vi "ESP Set and Get (SubVI).vi"(0 "ESP Config":T1={"COM Port Input"="COM8", "Manual Command"={"Device Type"="", "Instance"="", "Command"="", "Sub-Command"="", "Parameters (Seperate by :)"=""}, "Device Type"="e", "Instance"="a", "Use Manual Command"=TRUE, "Timeout [msec]"=1000, "Read/Write Wait [msec]"=25}, 5 "SET Table Ref":refnum<vi>, 7 "SET-GET Commands Ref":refnum<vi>) -> (4 "ESP Output":T2={"Write Command"="ea:DU:1", "Read String"="\u0006\u0001ea:00.000:00.000:00.036:00.004:AEA8\u0004", "Read Bytes"=12, "Bytes at Port"=12, "Response"="ea:00.000:00.000:00.036:00.004:AEA8", "ACK"=TRUE, "EOT"=TRUE, "NAK"=FALSE, "Parameters"=["00.000", "00.000", "00.036", "00.004"]}, 15 "ESP Error":errorcluster={"status"=FALSE, "code"=1073676294, "source"="VISA Read in ESP-D Read-Write (SubVI).vi->IO Board Evaluate.vi"})   [LabVIEW 2011]
panel:
  out "Error Output":errorcluster
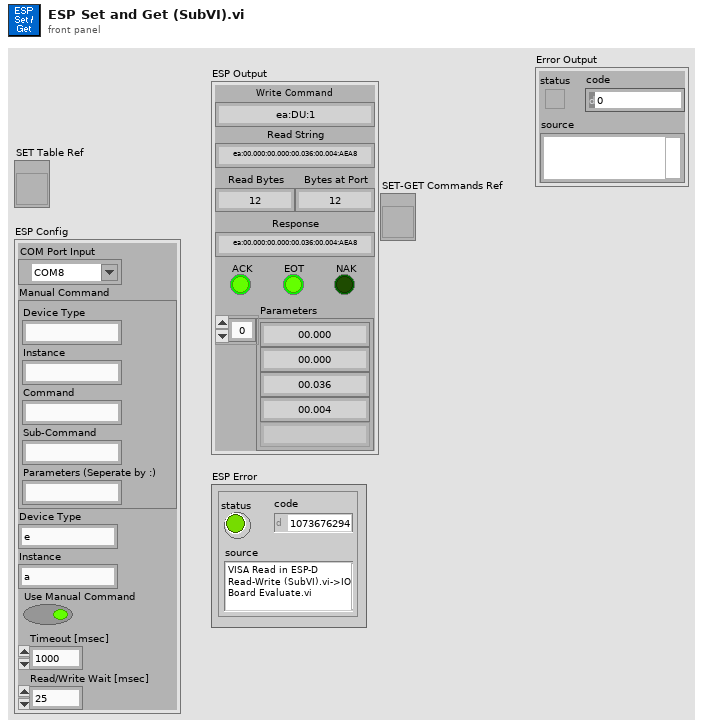
[diagram p1: front panel]
types:
  T1 = cluster{"COM Port Input":refnum<visa-resource-name>, "Manual Command":cluster{"Device Type":string, "Instance":string, "Command":string, "Sub-Command":string, "Parameters (Seperate by :)":string}, "Device Type":string, "Instance":string, "Use Manual Command":bool, "Timeout [msec]":u32, "Read/Write Wait [msec]":u32}
  T2 = cluster{"Write Command":string, "Read String":string, "Read Bytes":u32, "Bytes at Port":u32, "Response":string, "ACK":bool, "EOT":bool, "NAK":bool, "Parameters":string[]}
  T3 = cluster{"Device Type":string, "Instance":string, "Command":string, "Sub-Command":string, "Parameters (Seperate by :)":string}
  T4 = cluster{"CMD_Desc":string, "Param_Names":string[], "Param_Values":string[], "GET":bool, "SET":bool}
  T5 = cluster{"CMD_Desc":string, "Param_Names":string[], "Param_Values":string[], "SET":bool, "GET":bool}[]
  T6 = cluster{"CMD_Desc":string, "Param_Names":string[], "Param_Values":string[], "SET":bool, "GET":bool}
  T7 = cluster{"CMD_Desc":string, "Param_Names":string[], "Param_Values":string[], "GET":bool, "SET":bool}[]
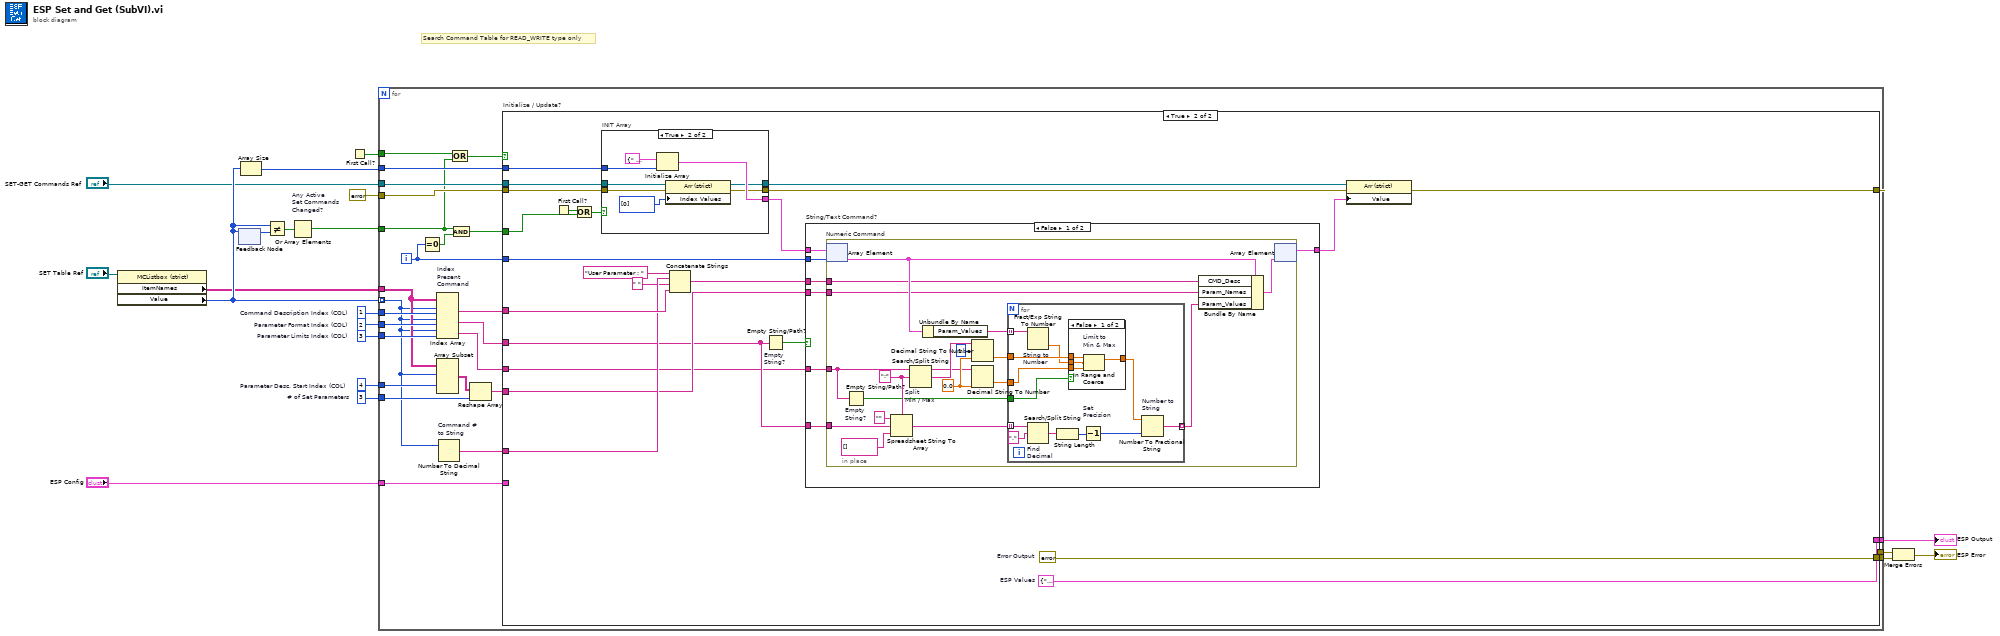
[diagram p0: block diagram]
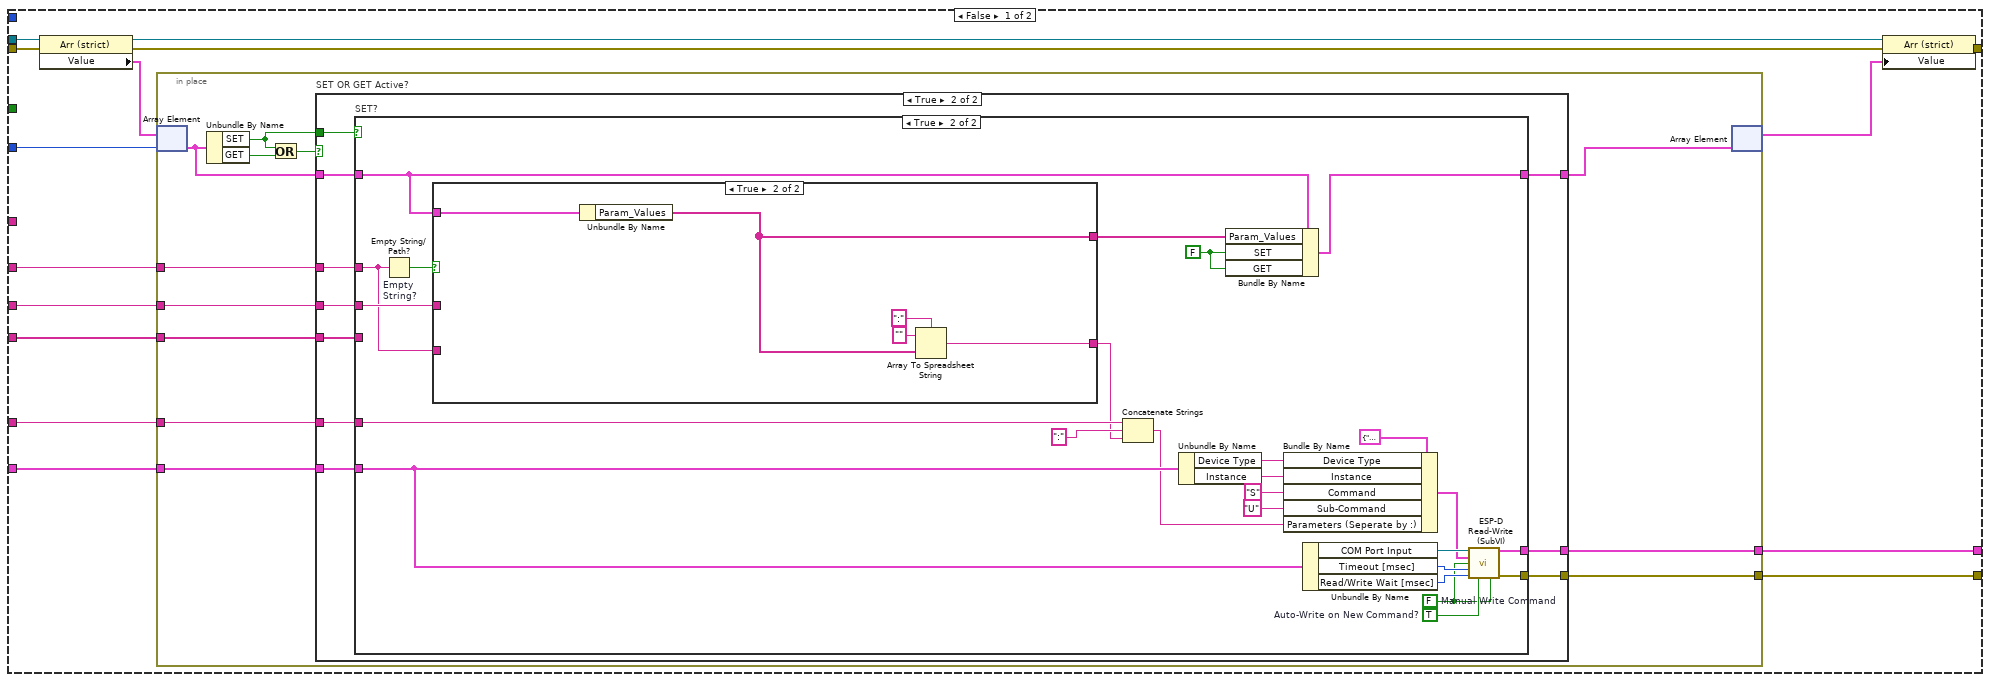
[diagram p2: hidden frame]
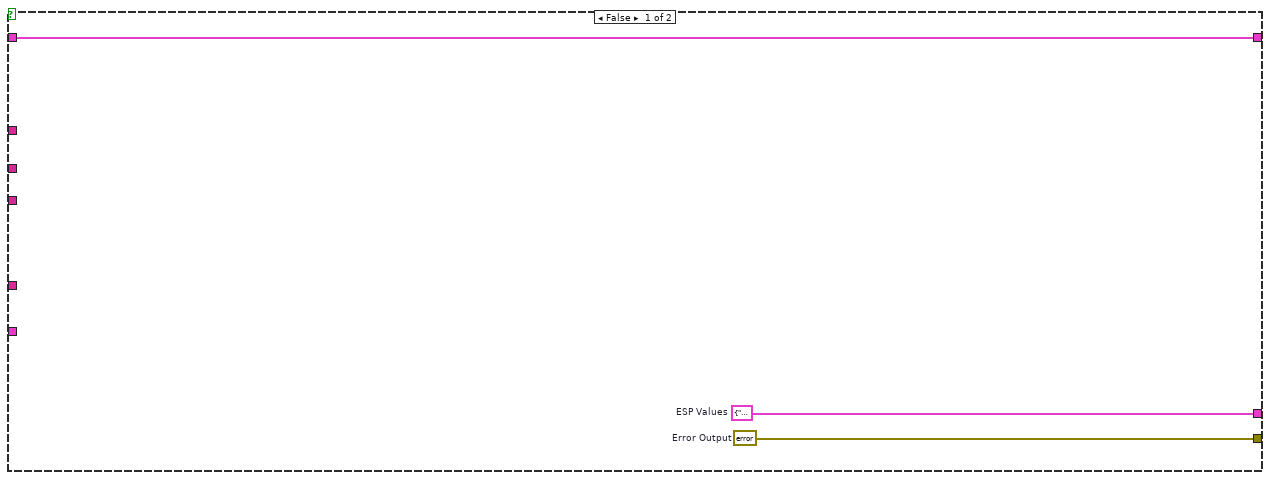
[diagram p3: hidden frame]
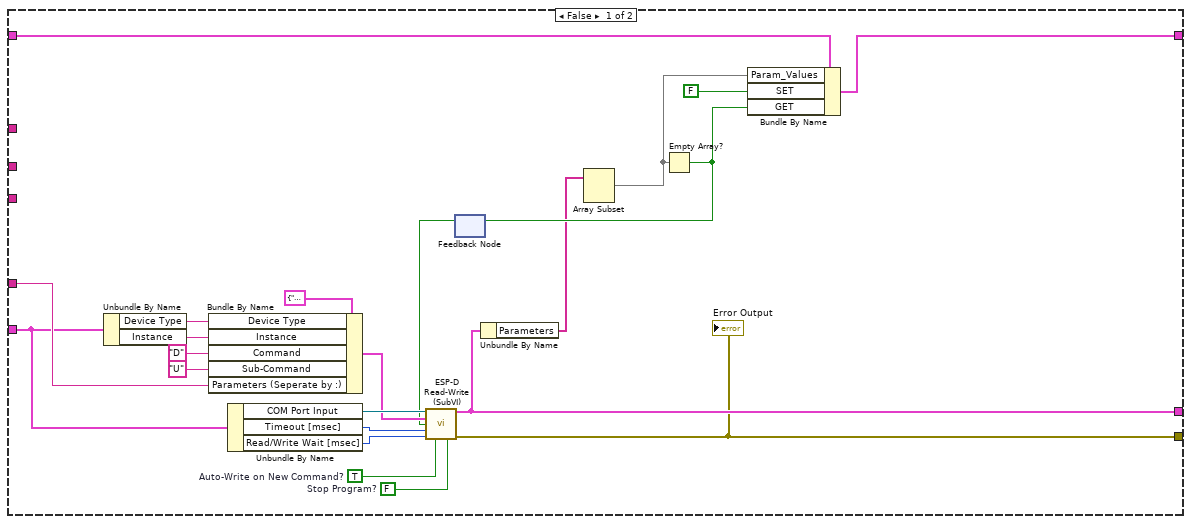
[diagram p4: hidden frame]
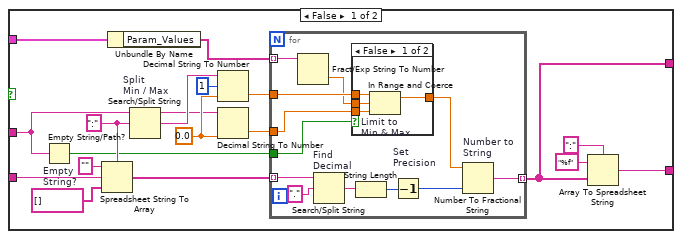
[diagram p5: hidden frame]
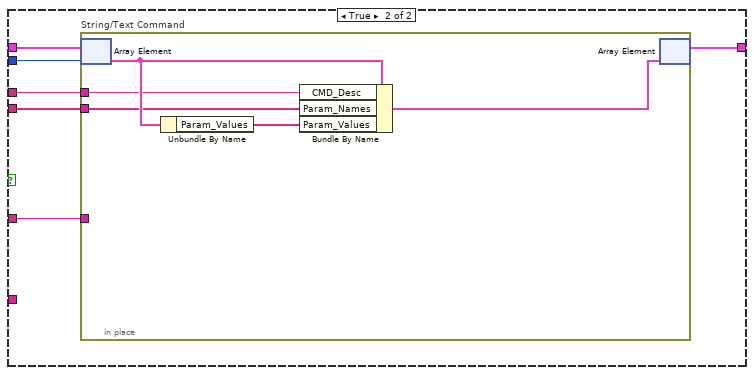
[diagram p8: hidden frame]
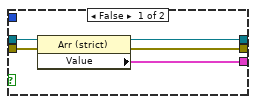
[diagram p9: hidden frame]
diagram:
  w8 = 1  # Command Description Index (COL)
  w5 = 3  # # of Set Parameters
  w6 = 4  # Parameter Desc. Start Index (COL)
  w4 = 3  # Parameter Limits Index (COL)
  w3 = 2  # Parameter Format Index (COL)
  # "Search Command Table for READ_WRITE type only"
  n1 = property class="MCListbox (strict)"(reference="SET Table Ref") -> ("ItemNames"=w9:string[][], "Value"=w14:i32[])  [unwired: 1 in, 2 out]
  n2 = feedback #1() -> (w13:i32[])  [unwired: 1 in]
  n3 = feedback-in #1(w14) -> ()
  n4 = Array Size(array=w14) -> (size(s)=w10:i32)
  n5 = Not Equal?(x=w14, y=w13) -> (x != y?=w12:bool[])
  n6 = Or Array Elements "Any Active\nSet Commands\nChanged?"(Boolean array=w12) -> (logical OR=w15:bool)
  n7 = First Call?() -> (First Call?: T/F=w11:bool)
  n8 = for {
    tunnel: "SET-GET Commands Ref" -> [w46]
    tunnel: w3 -> [w44]
    tunnel: w4 -> [w43]
    tunnel: w5 -> [w42]
    tunnel: w6 -> [w41]
    tunnel: errorcluster {"status"=FALSE, "code"=0, "source"=""} ("error in (no error)") -> [w40]
    tunnel: w8 -> [w39]
    tunnel: w14 -> [w24] mode=indexing
    tunnel: w9 -> [w34]
    tunnel: w10 -> [w33]
    tunnel: w11 -> [w28]
    tunnel: w15 -> [w27]
    tunnel: [w21] -> w16
    tunnel: [w26] -> w17
    tunnel: [w22] -> w18
    tunnel: "ESP Config" -> [w23]
    i -> [w31]
    n9 = Equal To 0?(x=w31) -> (x = 0?=w32:bool)
    n10 = Index Array "Index\nPresent\nCommand"(array=w34, index (row) #1=w24, index (col) #1=w39, index (row) #2=w24, index (col) #2=w44, index (row) #3=w24, index (col) #3=w43) -> (element #1=w37:string, element #2=w36:string, element #3=w35:string)
    n11 = Array Subset(array=w34, index (row)=w24, index (col)=w41) -> (w45:string[][])  [unwired: 2 in]
    n12 = Number To Decimal String "Command #\nto String"(number=w24) -> (decimal integer string=w25:string)  [unwired: 1 in]
    n13 = Or(x=w28, y=w27) -> (x .or. y?=w30:bool)
    n14 = And(x=w27, y=w32) -> (x .and. y?=w29:bool)
    n15 = Reshape Array(w45, w42) -> (w38:string[])
    n16 = case "Initialize / Update?" shown="True" w30 {
      tunnel: w46 -> [w61 w197]
      tunnel: w37 -> [_ w196]
      tunnel: w40 -> [w60 w195]
      tunnel: w31 -> [w53 w193]
      tunnel: [w57 w194] -> w26
      tunnel: w25 -> [w51 w192]
      tunnel: w38 -> [w47 w191]
      tunnel: w36 -> [w55 w190]
      tunnel: w35 -> [w56 w189]
      tunnel: w33 -> [_ w188]
      tunnel: w29 -> [_ w187]
      tunnel: w23 -> [w52 _]
      tunnel: [w50 w177] -> w22
      tunnel: [w49 w176] -> w21
      frame False {
        n17 = property class="Arr (strict)"(reference=w61, error in=w60) -> (reference out=w59:refnum<vi>, error out=w58:errorcluster, "Value"=w54:T5)
        n18 = in-place {
          in-place-border: w56 -> [w73]
          in-place-border: w55 -> [w72]
          in-place-border: w52 -> [w67]
          in-place-border: w51 -> [w66]
          in-place-border: [w65] -> w50
          in-place-border: [w64] -> w49
          in-place-border: w47 -> [w62]
          n19 = in-place-array #2(w54, w53) -> (w68:T6)
          n20 = Unbundle By Name(w68) -> ("SET"=w71:bool, "GET"=w70:bool)
          n21 = Or(x=w71, y=w70) -> (x .or. y?=w69:bool)
          n22 = case "SET OR GET Active?" shown="True" w69 {
            tunnel: w73 -> [_ w86]
            tunnel: w72 -> [_ w78]
            tunnel: w71 -> [_ w85]
            tunnel: w68 -> [w74 w80]
            tunnel: w67 -> [_ w84]
            tunnel: w66 -> [_ w83]
            tunnel: [w75 w82] -> w65
            tunnel: [w76 w81] -> w64
            tunnel: [w74 w79] -> w63
            tunnel: w62 -> [_ w77]
            frame False {
              w75 = T2 {"Write Command"="", "Read String"="", "Read Bytes"=0, "Bytes at Port"=0, "Response"="", "ACK"=FALSE, "EOT"=FALSE, "NAK"=FALSE, "Parameters"=[]}  # ESP Values
              w76 = errorcluster {"status"=FALSE, "code"=0, "source"=""}  # Error Output
            }
            frame True {
              n23 = case "SET?" shown="True" w85 {
                tunnel: w86 -> [_ w133]
                tunnel: w78 -> [_ w114]
                tunnel: w84 -> [w105 w128]
                tunnel: w83 -> [w106 w131]
                tunnel: [w104 w118] -> w82
                tunnel: [w103 w117] -> w81
                tunnel: w80 -> [w108 w109]
                tunnel: [w107 w111] -> w79
                tunnel: w77 -> [_ _]
                frame False {
                  w92 = FALSE  # Stop Program?
                  w94 = TRUE  # Auto-Write on New Command?
                  n24 = Unbundle By Name(w105) -> ("Device Type"=w101:string, "Instance"=w100:string)
                  n25 = Bundle By Name(cluster=T3 {"Device Type"="", "Instance"="", "Command"="", "Sub-Command"="", "Parameters (Seperate by :)"=""}, "Device Type"=w101, "Instance"=w100, "Command"="D", "Sub-Command"="U", "Parameters (Seperate by :)"=w106) -> (w93:T3)
                  n26 = Unbundle By Name(w105) -> ("COM Port Input"=w97:refnum<visa-resource-name>, "Timeout [msec]"=w95:u32, "Read/Write Wait [msec]"=w96:u32)
                  n27 = feedback #3() -> (w91:bool)  [unwired: 1 in]
                  n28 = call "ESP-D Read-Write (SubVI).vi"("COM Port Input"=w97, "Command Input"=w93, "Manual Write Command"=w91, "Timeout (ms)"=w95, "Write/Read Wait (ms)"=w96, "Auto-Write on New Command?"=w94, "Stop Program?"=w92) -> ("ESP Values"=w104:T2, "Error Output"=w103:errorcluster)  [unwired: 7 in]
                  "Error Output" <- w103
                  n29 = Unbundle By Name(w104) -> ("Parameters"=w88:string[])
                  n30 = Array Subset(array=w88) -> (w87:string[])  [unwired: 2 in]
                  n31 = Empty Array?(array=w87) -> (empty?=w90:bool)
                  n32 = feedback-in #3(w90) -> ()
                  n33 = Bundle By Name(cluster=w108, "Param_Values"=w87, "SET"=FALSE, "GET"=w90) -> (w107:T6)
                }
                frame True {
                  w112 = FALSE
                  w120 = TRUE  # Auto-Write on New Command?
                  w119 = FALSE  # Manual Write Command
                  n34 = Empty String/Path? "Empty\nString?"(string/path=w114) -> (empty?=w113:bool)
                  n35 = case shown="True" w113 {
                    tunnel: [w152 w174] -> w130
                    tunnel: w114 -> [w151 _]
                    tunnel: w133 -> [w150 _]
                    tunnel: w109 -> [w135 w173]
                    tunnel: [w134 w170] -> w110
                    frame False {
                      w142 = 0.0
                      w149 = ":" ("delimiter (Tab)")
                      n36 = Empty String/Path? "Empty\nString?"(string/path=w150) -> (empty?=w136:bool)
                      n37 = Spreadsheet String To Array(delimiter (Tab)=w149, format string="", spreadsheet string=w151, array type (2D Dbl)=string[] []) -> (array=w147:string[])
                      n38 = Unbundle By Name(w135) -> ("Param_Values"=w138:string[])
                      n39 = Search/Split String "Split\nMin / Max"(string=w150, search string/char (-)=w149) -> (substring before match=w141:string, match + rest of string=w143:string)  [unwired: 1 in, 1 out]
                      n40 = Decimal String To Number(string=w143, offset=1, default (0L)=w142) -> (number=w145:dbl)  [unwired: 1 out]
                      n41 = Decimal String To Number(string=w141, default (0L)=w142) -> (number=w146:dbl)  [unwired: 1 in, 1 out]
                      n42 = for {
                        tunnel: w147 -> [w160] mode=indexing
                        tunnel: w145 -> [w162]
                        tunnel: w146 -> [w163]
                        tunnel: [w156] -> w134 mode=indexing
                        tunnel: w138 -> [w154] mode=indexing
                        tunnel: w136 -> [w153]
                        n43 = Fract/Exp String To Number(string=w154) -> (number=w161:dbl)  [unwired: 3 in, 1 out]
                        n44 = Search/Split String "Find\nDecimal"(string=w160, search string/char (-)=".") -> (match + rest of string=w159:string)  [unwired: 1 in, 2 out]
                        n45 = case shown="False" w153 {
                          tunnel: w163 -> [w168 _]
                          tunnel: w162 -> [w167 _]
                          tunnel: w161 -> [w166 w169]
                          tunnel: [w165 w169] -> w155
                          frame False {
                            n46 = In Range and Coerce "Limit to\nMin & Max"(upper limit=w167, x=w166, lower limit=w168) -> (coerced(x)=w165:dbl)  [unwired: 1 out]
                          }
                          frame True {
                          }
                        }
                        n47 = String Length(string=w159) -> (length=w157:i32)
                        n48 = Decrement "Set\nPrecision"(x=w157) -> (x-1=w158:i32)
                        n49 = Number To Fractional String "Number to\nString"(number=w155, precision (6)=w158) -> (F-format string=w156:string)  [unwired: 2 in]
                      }
                      n50 = Array To Spreadsheet String(delimiter (Tab)=":", array=w134, 3:"%f" ("format string")) -> (spreadsheet string=w152:string)
                    }
                    frame True {
                      n51 = Unbundle By Name(w173) -> ("Param_Values"=w170:string[])
                      n52 = Array To Spreadsheet String(delimiter (Tab)=":", array=w170, 3:"" ("format string")) -> (spreadsheet string=w174:string)
                    }
                  }
                  n53 = Concatenate Strings(w131, ":" ("delimiter (Tab)"), w130) -> (w116:string)
                  n54 = Unbundle By Name(w128) -> ("Device Type"=w127:string, "Instance"=w126:string)
                  n55 = Bundle By Name(cluster=w109, "Param_Values"=w110, "SET"=w112, "GET"=w112) -> (w111:T6)
                  n56 = Bundle By Name(cluster=T3 {"Device Type"="", "Instance"="", "Command"="", "Sub-Command"="", "Parameters (Seperate by :)"=""}, "Device Type"=w127, "Instance"=w126, "Command"="S", "Sub-Command"="U", "Parameters (Seperate by :)"=w116) -> (w115:T3)
                  n57 = Unbundle By Name(w128) -> ("COM Port Input"=w123:refnum<visa-resource-name>, "Timeout [msec]"=w121:u32, "Read/Write Wait [msec]"=w122:u32)
                  n58 = call "ESP-D Read-Write (SubVI).vi"("COM Port Input"=w123, "Command Input"=w115, "Manual Write Command"=w119, "Timeout (ms)"=w121, "Write/Read Wait (ms)"=w122, "Auto-Write on New Command?"=w120, "Stop Program?"=w119) -> ("ESP Values"=w118:T2, "Error Output"=w117:errorcluster)  [unwired: 7 in]
                }
              }
            }
          }
          n59 = in-place-array #2(w63) -> (w48:T5)  [unwired: 1 out]
        }
        n60 = property class="Arr (strict)"(reference=w59, error in=w58, "Value"=w48) -> (error out=w57:errorcluster)  [unwired: 1 out]
      }
      frame True {
        w177 = T2 {"Write Command"="", "Read String"="", "Read Bytes"=0, "Bytes at Port"=0, "Response"="", "ACK"=FALSE, "EOT"=FALSE, "NAK"=FALSE, "Parameters"=[]}  # ESP Values
        w176 = errorcluster {"status"=FALSE, "code"=0, "source"=""}  # Error Output
        n61 = First Call?() -> (First Call?: T/F=w178:bool)
        n62 = Or(x=w178, y=w187) -> (x .or. y?=w179:bool)
        n63 = case "INIT Array" shown="True" w179 {
          tunnel: [w252 w264] -> w185
          tunnel: w188 -> [_ w263]
          tunnel: w197 -> [w256 w260]
          tunnel: w195 -> [w255 w258]
          tunnel: [w254 w259] -> w182
          tunnel: [w253 w257] -> w181
          frame False {
            n64 = property class="Arr (strict)"(reference=w256, error in=w255) -> (reference out=w254:refnum<vi>, error out=w253:errorcluster, "Value"=w252:T5)
          }
          frame True {
            n65 = Initialize Array(T4 {"CMD_Desc"=" ", "Param_Names"=["", "", " "], "Param_Values"=["", "", " "], "GET"=FALSE, "SET"=FALSE} ("Cluster 2"), w263) -> (w264:T7)
            n66 = property class="Arr (strict)"(reference=w260, error in=w258, "Index Values"=u32[] [0]) -> (reference out=w259:refnum<vi>, error out=w257:errorcluster)
          }
        }
        n67 = Concatenate Strings("User Parameter : " ("string"), w192, " ", w196) -> (w183:string)
        n68 = Empty String/Path? "Empty\nString?"(string/path=w190) -> (empty?=w180:bool)
        n69 = case "String/Text Command?" shown="False" w180 {
          tunnel: w190 -> [w204 _]
          tunnel: w189 -> [w203 w246]
          tunnel: w185 -> [w202 w245]
          tunnel: w193 -> [w201 w244]
          tunnel: w191 -> [w200 w243]
          tunnel: [w199 w242] -> w184
          tunnel: w183 -> [w198 w241]
          frame False {
            n70 = in-place "Numeric Command" {
              in-place-border: w204 -> [w213]
              in-place-border: w203 -> [w206]
              in-place-border: w198 -> [w210]
              in-place-border: w200 -> [w209]
              w217 = 0.0
              w223 = ":" ("delimiter (Tab)")
              n71 = in-place-array #4(w202, w201) -> (w211:T4)
              n72 = Empty String/Path? "Empty\nString?"(string/path=w206) -> (empty?=w205:bool)
              n73 = Spreadsheet String To Array(delimiter (Tab)=w223, format string="", spreadsheet string=w213, array type (2D Dbl)=string[] []) -> (array=w222:string[])
              n74 = Search/Split String "Split\nMin / Max"(string=w206, search string/char (-)=w223) -> (substring before match=w216:string, match + rest of string=w218:string)  [unwired: 1 in, 1 out]
              n75 = Unbundle By Name(w211) -> ("Param_Values"=w212:string[])
              n76 = Decimal String To Number(string=w218, offset=1, default (0L)=w217) -> (number=w220:dbl)  [unwired: 1 out]
              n77 = Decimal String To Number(string=w216, default (0L)=w217) -> (number=w221:dbl)  [unwired: 1 in, 1 out]
              n78 = for {
                tunnel: w222 -> [w231] mode=indexing
                tunnel: w220 -> [w233]
                tunnel: w221 -> [w234]
                tunnel: [w227] -> w208 mode=indexing
                tunnel: w212 -> [w225] mode=indexing
                tunnel: w205 -> [w224]
                n79 = Fract/Exp String To Number "String to\nNumber"(string=w225) -> (number=w232:dbl)  [unwired: 3 in, 1 out]
                n80 = Search/Split String "Find\nDecimal"(string=w231, search string/char (-)=".") -> (match + rest of string=w230:string)  [unwired: 1 in, 2 out]
                n81 = String Length(string=w230) -> (length=w228:i32)
                n82 = case shown="False" w224 {
                  tunnel: w234 -> [w239 _]
                  tunnel: w233 -> [w238 _]
                  tunnel: w232 -> [w237 w240]
                  tunnel: [w236 w240] -> w226
                  frame False {
                    n83 = In Range and Coerce "Limit to\nMin & Max"(upper limit=w238, x=w237, lower limit=w239) -> (coerced(x)=w236:dbl)  [unwired: 1 out]
                  }
                  frame True {
                  }
                }
                n84 = Decrement "Set\nPrecision"(x=w228) -> (x-1=w229:i32)
                n85 = Number To Fractional String "Number to\nString"(number=w226, precision (6)=w229) -> (F-format string=w227:string)  [unwired: 2 in]
              }
              n86 = Bundle By Name(cluster=w211, "CMD_Desc"=w210, "Param_Names"=w209, "Param_Values"=w208) -> (w207:T4)
              n87 = in-place-array #4(w207) -> (w199:T7)  [unwired: 1 out]
            }
          }
          frame True {
            n88 = in-place "String/Text Command" {
              in-place-border: w246 -> [_]
              in-place-border: w241 -> [w250]
              in-place-border: w243 -> [w249]
              n89 = in-place-array #5(w245, w244) -> (w251:T4)
              n90 = Unbundle By Name(w251) -> ("Param_Values"=w247:string[])
              n91 = Bundle By Name(cluster=w251, "CMD_Desc"=w250, "Param_Names"=w249, "Param_Values"=w247) -> (w248:T4)
              n92 = in-place-array #5(w248) -> (w242:T7)  [unwired: 1 out]
            }
          }
        }
        n93 = property class="Arr (strict)"(reference=w182, error in=w181, "Value"=w184) -> (error out=w194:errorcluster)  [unwired: 1 out]
      }
    }
  }
  "ESP Output" <- w18
  n94 = Merge Errors(w17, w16) -> (→"ESP Error":errorcluster)
